vi "Read Network.vi"(8 "error in (no error)":errorcluster, 11 "Sensor Engine Datas in":T1[](array[typedef]) {"MM Frames"."payload" format="%x"; "MM Frames"."timestamp" format="%<%.7X\n%x>T"; "MM Frames"."type" items=["FlexRay Data"=32, "FlexRay Null"=33, "FlexRay Symbol"=34, "Log Trigger"=225, "Start Trigger"=226]; "MM Frames"."cycle count" max=63 step=1}) -> (0 "error out":errorcluster, 1 "signal data":dbl[](array[numeric]), 3 "Sensor Engine Datas out":T1[](array[typedef]) {"MM Frames"."payload" format="%x"; "MM Frames"."timestamp" format="%<%.7X\n%x>T"; "MM Frames"."type" items=["FlexRay Data"=32, "FlexRay Null"=33, "FlexRay Symbol"=34, "Log Trigger"=225, "Start Trigger"=226]; "MM Frames"."cycle count" max=63 step=1}, 5 "Array":i32[](array[numeric]))   [LabVIEW 2018, in "MM.lvlib"]
uses:
  MM.lvlib
  Sensor Engine Data.ctl
  Shared/Protocol.ctl
  Shared/Sensor Name.ctl
  <vilib>/xnet/xnet.llb/XNET Frame FlexRay.ctl
  <vilib>/xnet/xnet.llb/XNET Frame Type FlexRay.ctl
  <vilib>/xnet/xnet.llb/XNET Convert (Frame FlexRay to Signal).vi
  Shared/Vires VTD Shared.lvlib
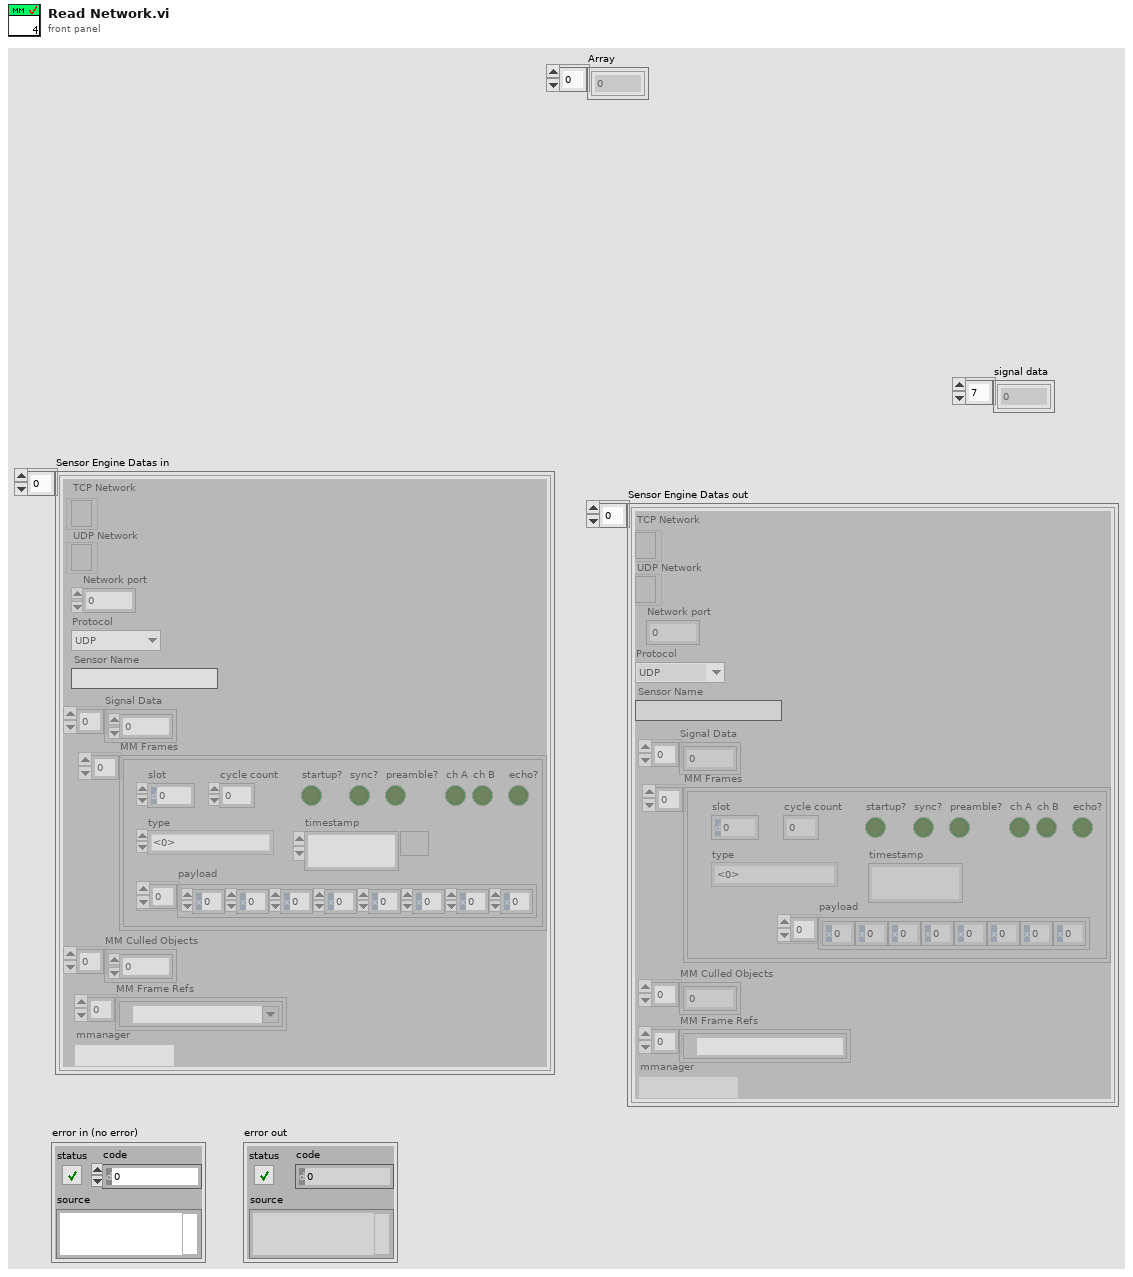
[diagram p1: front panel]
types:
  T1 = typedef "MM.lvlib/Sensor Engine Data.ctl" = cluster{"TCP Network":refnum<k5>, "UDP Network":refnum<k16>, "Network port":i32, "Protocol":T2, "Sensor Name":T3, "Signal Data":dbl[], "MM Frames":T4[], "MM Culled Objects":i32[], "MM Frame Refs":refnum<k21>[], "mmanager":path}
  T2 = typedef "Vires VTD Shared.lvlib/Protocol.ctl" = enum16{"UDP", "TCP"}
  T3 = typedef "Vires VTD Shared.lvlib/Sensor Name.ctl" = string
  T4 = typedef "XNET Frame FlexRay.ctl" = cluster{"timestamp":timestamp, "payload":u8[], "slot":u16, "type":T5, "cycle count":u8, "startup?":bool, "sync?":bool, "preamble?":bool, "ch A":bool, "ch B":bool, "echo?":bool}
  T5 = typedef "XNET Frame Type FlexRay.ctl" = u8
  T6 = enum16{"Standard", "Buffered", "CRLF", "Immediate"}
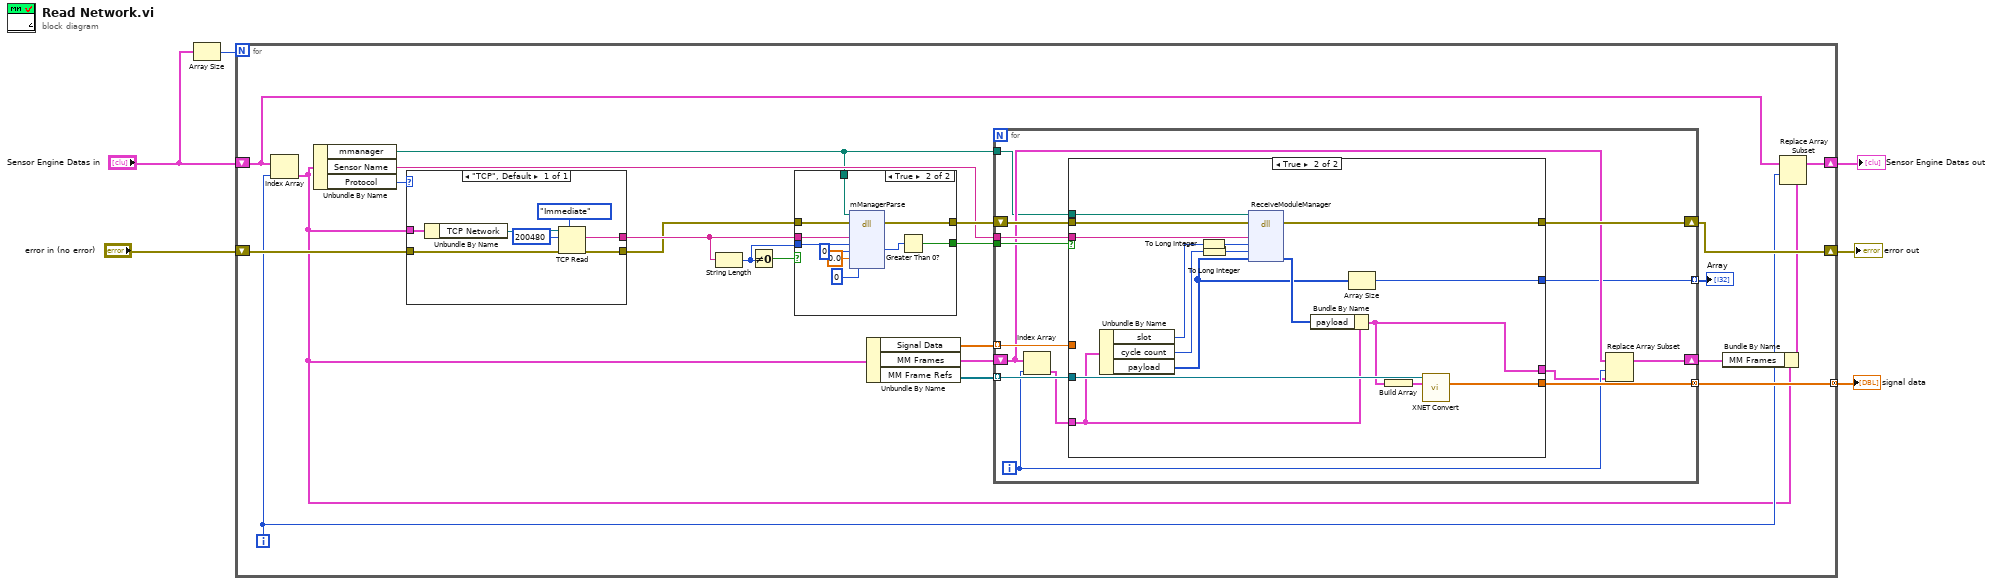
[diagram p0: block diagram]
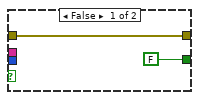
[diagram p3: hidden frame]
diagram:
  n1 = Array Size(array="Sensor Engine Datas in") -> (size(s)=w2:i32)
  n2 = for {
    N: w2 -> [_]
    shift-right: [w20] -> w5
    shift-left: "error in (no error)" -> [w27]
    tunnel: [w18] -> w4 mode=concatenating
    shift-right: [w14] -> w3
    shift-left: "Sensor Engine Datas in" -> [w13]
    i -> [w12]
    n3 = Index Array(array=w13, index=w12) -> (element=w11:T1)
    n4 = Unbundle By Name(w11) -> ("mmanager"=w7:path, "Sensor Name"=w19:T3, "Protocol"=w28:T2)
    n5 = case shown="\"TCP\", Default" w28 {
      tunnel: w27 -> [w79]
      tunnel: [w77] -> w23
      tunnel: [w76] -> w24
      tunnel: w11 -> [w74]
      frame "TCP", Default {
        n6 = Unbundle By Name(w74) -> ("TCP Network"=w73:refnum<k5>)
        n7 = TCP Read(connection ID=w73, bytes to read=200480, error in (no error)=w79, 7:T6."Immediate" ("mode (standard)")) -> (data out=w76:string, error out=w77:errorcluster)  [unwired: 1 in, 1 out]
      }
    }
    n8 = String Length(string=w24) -> (length=w26:i32)
    n9 = Not Equal To 0?(x=w26) -> (x != 0?=w25:bool)
    n10 = case shown="True" w25 {
      tunnel: w23 -> [w62 w72]
      tunnel: [w62 w71] -> w22
      tunnel: w24 -> [_ w70]
      tunnel: [FALSE w67] -> w21
      tunnel: w26 -> [_ w66]
      tunnel: w7 -> [_ w63]
      frame False {
      }
      frame True {
        n11 = dll-call lib="ModuleManager.dlls" fn="mManagerParse"(path in=w63, error in=w72, "RDBmessage"=w70, "size"=w66, "valid"=u8 0, "simTime"=0.0, "simFrame"=0) -> (error out=w71:errorcluster, "valid"=w68:u8)  [unwired: 6 in, 1 out]
        n12 = Greater Than 0?(x=w68) -> (x > 0?=w67:bool)
      }
    }
    n13 = Unbundle By Name(w11) -> ("Signal Data"=w15:dbl[], "MM Frames"=w17:T4[], "MM Frame Refs"=w16:refnum<k21>[])
    n14 = for {
      tunnel: w21 -> [w41]
      tunnel: w19 -> [w39]
      tunnel: [w38] -> w18 mode=concatenating
      shift-right: [w40] -> w20
      shift-left: w22 -> [w42]
      tunnel: w16 -> [w36] mode=indexing
      tunnel: w15 -> [w37] mode=indexing
      shift-right: [w34] -> w9
      shift-left: w17 -> [w33]
      tunnel: [w30] -> w8 mode=indexing
      tunnel: w7 -> [w29]
      i -> [w32]
      n15 = Index Array(array=w33, index=w32) -> (element=w35:T4)
      n16 = case shown="True" w41 {
        tunnel: w42 -> [w44 w60]
        tunnel: [w44 w59] -> w40
        tunnel: w39 -> [_ w58]
        tunnel: [_ w57] -> w38
        tunnel: w37 -> [_ _]
        tunnel: w36 -> [_ w54]
        tunnel: w35 -> [w43 w53]
        tunnel: [w43 w50] -> w31
        tunnel: [_ w46] -> w30
        tunnel: w29 -> [_ w45]
        frame False {
        }
        frame True {
          n17 = Unbundle By Name(w53) -> ("slot"=w52:u16, "cycle count"=w51:u8, "payload"=w47:u8[])
          n18 = To Long Integer(number=w52) -> (32bit integer=w49:i32)
          n19 = To Long Integer(number=w51) -> (32bit integer=w48:i32)
          n20 = dll-call lib="ModuleManager.dll" fn="ReceiveModuleManager"(path in=w45, error in=w60, "SensorName"=w58, "pkID"=w49, "Element"=w48, "Item"=w47) -> (error out=w59:errorcluster, "Item"=w56:u8[])  [unwired: 5 in, 1 out]
          n21 = Bundle By Name(cluster=w53, "payload"=w56) -> (w50:T4)
          n22 = Array Size(array=w47) -> (size(s)=w46:i32)
          n23 = Build Array(w50) -> (w55:T4[])
          n24 = call-poly <vilib>:"XNET Convert.vi"("session in"=w54, "frame data"=w55) -> ("signal data"=w57:dbl[])  [unwired: 11 in, 2 out]
        }
      }
      n25 = Replace Array Subset(array=w33, new element=w31, index=w32) -> (w34:T4[])
    }
    "Array" <- w8
    n26 = Bundle By Name(cluster=w11, "MM Frames"=w9) -> (w10:T1)
    n27 = Replace Array Subset(array=w13, new element=w10, index=w12) -> (w14:T1[])
  }
  "error out" <- w5
  "signal data" <- w4
  "Sensor Engine Datas out" <- w3
